vi "Delete alias files.vi"(8 "error in":errorcluster, 11 "Directory Path":path) -> (0 "error out":errorcluster)   [LabVIEW 2021, in "Plugin Generator.lvlib"]
uses:
  Plugin Generator.lvlib
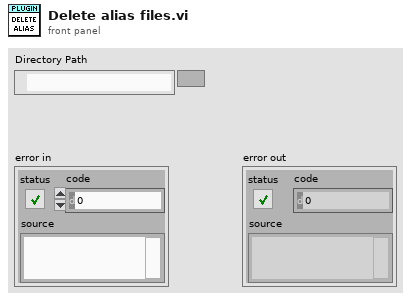
[diagram p1: front panel]
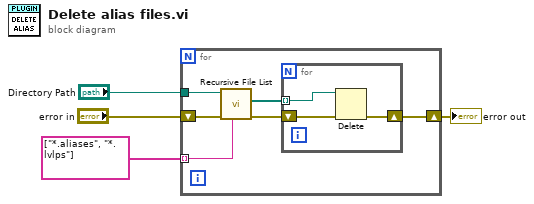
[diagram p0: block diagram]
diagram:
  n1 = for {
    tunnel: "Directory Path" -> [w10]
    tunnel: string[] ["*.aliases", "*.lvlps"] -> [w7] mode=indexing
    shift-right: [w6] -> w1
    shift-left: "error in" -> [w5]
    n2 = call <vilib>:"Recursive File List.vi"("pattern"=w7, "error in (no error)"=w5, "Folder Path"=w10) -> ("error out"=w8:errorcluster, "All Files in Dir"=w9:path[])  [unwired: 4 in, 3 out]
    n3 = for {
      tunnel: w9 -> [w13] mode=indexing
      shift-right: [w11] -> w6
      shift-left: w8 -> [w12]
      n4 = Delete(path (use dialog)=w13, error in=w12) -> (error out=w11:errorcluster)  [unwired: 3 in, 2 out]
    }
  }
  "error out" <- w1
